vi "Add VI Template to Library.vi"(7 "Template VI Refnum":refnum<vi>, 8 "error in":errorcluster, 9 "VI Name":string, 10 "Custom Device Folder":path, 11 "Custom Device Library in":refnum<vi>) -> (0 "error out":errorcluster, 1 "VI Path out":path, 2 "Custom Device Folder out":path, 3 "Custom Device Library out":refnum<vi>)   [LabVIEW 2019, in "Custom Device Template Tool.lvlib"]
uses:
  Custom Device Template Tool.lvlib
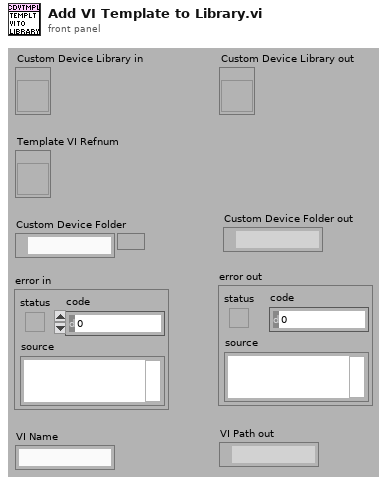
[diagram p1: front panel]
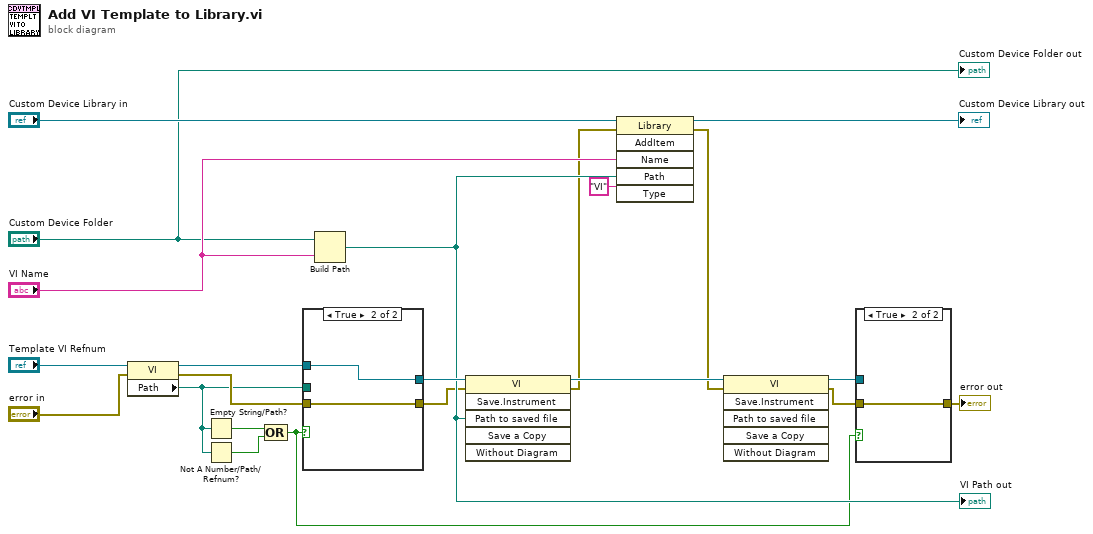
[diagram p0: block diagram]
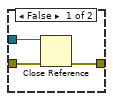
[diagram p2: hidden frame]
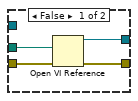
[diagram p3: hidden frame]
diagram:
  n1 = property class="VI"(reference="Template VI Refnum", error in="error in") -> (reference out=w4:refnum<vi>, error out=w8:errorcluster, "Path"=w3:path)
  n2 = Empty String/Path?(string/path=w3) -> (empty?=w5:bool)
  n3 = Not A Number/Path/Refnum?(number/path/refnum=w3) -> (NaN/Path/Refnum?=w2:bool)
  n4 = Compound Arithmetic op=OR(w5, w2) -> (w1:bool)
  n5 = case shown="True" w1 {
    tunnel: [w26 w28] -> w16
    tunnel: w8 -> [w25 w27]
    tunnel: [w24 w27] -> w7
    tunnel: w3 -> [w23 _]
    tunnel: w4 -> [_ w28]
    frame False {
      n6 = Open VI Reference(vi path=w23, error in (no error)=w25) -> (vi reference=w26:refnum<vi>, error out=w24:errorcluster)  [unwired: 4 out]
    }
    frame True {
    }
  }
  n7 = Build Path(base path="Custom Device Folder", name or relative path="VI Name") -> (appended path=w15:path)
  "VI Path out" <- w15
  n8 = invoke class="VI" method="Save.Instrument"(reference=w16, error in=w7, "Path to saved file"=w15) -> (reference out=w18:refnum<vi>, error out=w6:errorcluster)  [unwired: 3 in, 4 out]
  n9 = invoke class="Library" method="AddItem"(reference="Custom Device Library in", error in=w6, "Name"="VI Name", "Path"=w15, "Type"="VI") -> (reference out=→"Custom Device Library out":refnum<vi>, error out=w17:errorcluster)  [unwired: 1 in, 4 out]
  n10 = invoke class="VI" method="Save.Instrument"(reference=w18, error in=w17) -> (reference out=w20:refnum<vi>, error out=w21:errorcluster)  [unwired: 4 in, 4 out]
  n11 = case shown="True" w1 {
    tunnel: [w31 w32] -> w22
    tunnel: w21 -> [w30 w32]
    tunnel: w20 -> [w29 _]
    frame False {
      n12 = Close Reference(reference=w29, error in (no error)=w30) -> (error out=w31:errorcluster)
    }
    frame True {
    }
  }
  "error out" <- w22
  "Custom Device Folder out" <- "Custom Device Folder"
